vi "CmdConsole.Kill.vi"(8 "error in":errorcluster, 11 "CmdConsole in":refnum<class "CmdConsole.lvclass">) -> (0 "error out":errorcluster, 3 "CmdConsole out":refnum<class "CmdConsole.lvclass">)   [LabVIEW 2018, in "CmdConsole.lvclass"]
uses:
  CmdConsole.lvclass
  CmdConsole.lvclass/CmdConsole.ctl
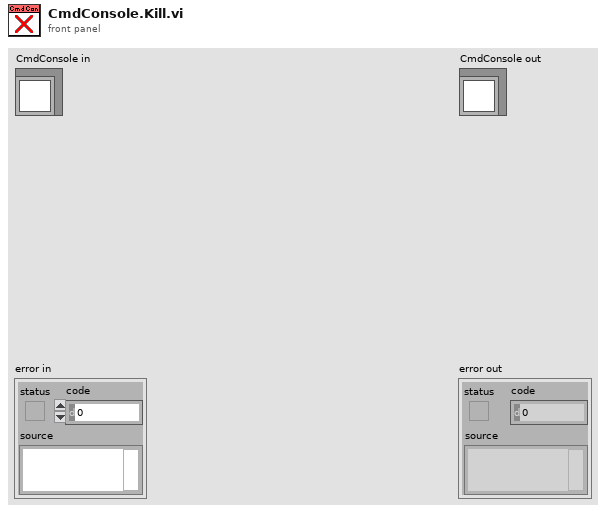
[diagram p1: front panel]
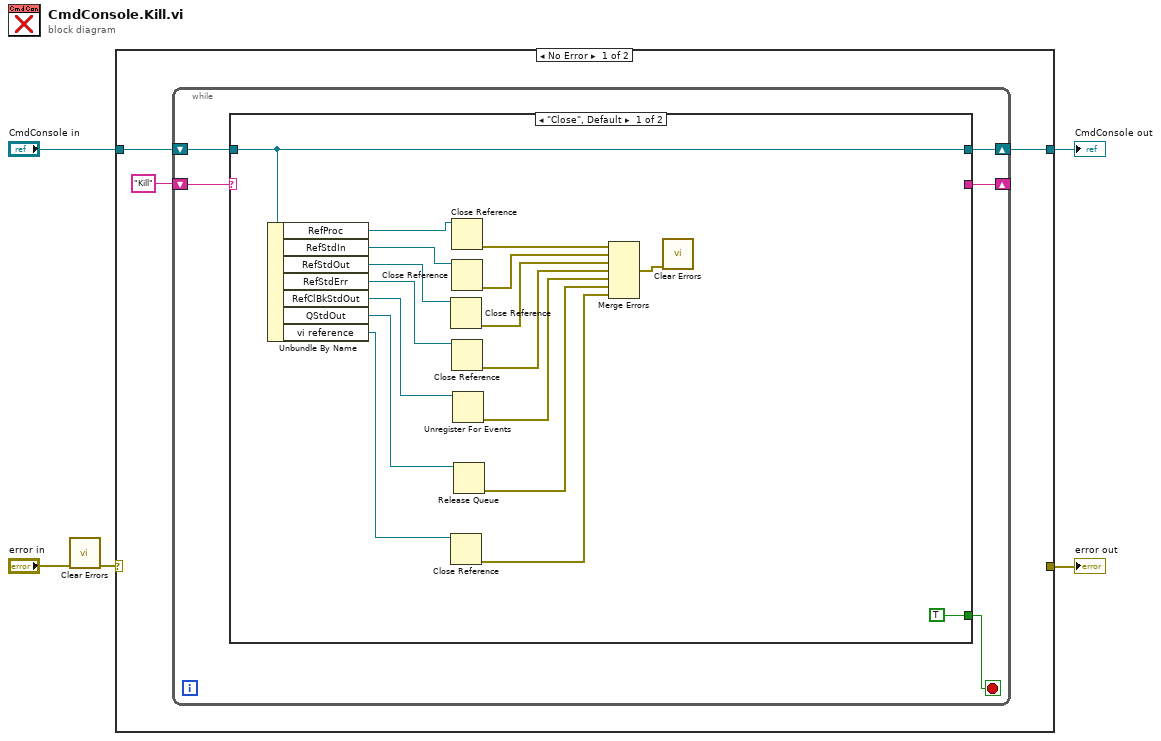
[diagram p0: block diagram]
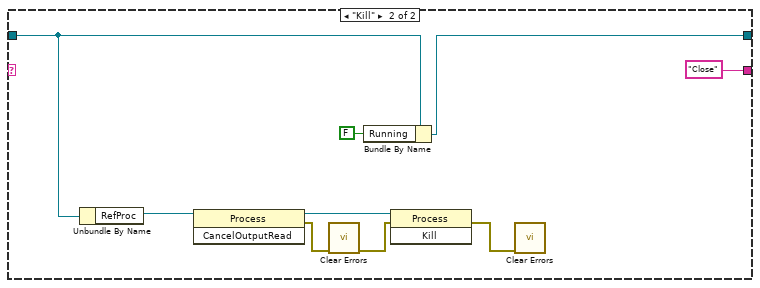
[diagram p2: hidden frame]
diagram:
  n1 = call <vilib>:"Clear Errors.vi"("error in (no error)"="error in") -> ("error out"=w2:errorcluster)  [unwired: 5 in, 1 out]
  n2 = case shown="No Error" w2 {
    selector: w2 -> [_ w41]
    tunnel: [_ w41] -> w5
    tunnel: [w7 w40] -> w3
    tunnel: "CmdConsole in" -> [w8 w40]
    frame No Error {
      n3 = while {
        shift-right: [w12] -> w7
        shift-left: w8 -> [w11]
        shift-right: [w13] -> _
        shift-left: "Kill" -> [w10]
        stop <- w9 stop-if-true
        n4 = case shown="\"Close\", Default" w10 {
          tunnel: w11 -> [w16 w33]
          tunnel: [_ "Close"] -> w13
          tunnel: [w16 w32] -> w12
          tunnel: [TRUE _] -> w9
          frame "Close", Default {
            n5 = Unbundle By Name(w16) -> ("RefProc"=w23:refnum<k24>, "RefStdIn"=w22:refnum<k24>, "RefStdOut"=w21:refnum<k24>, "RefStdErr"=w20:refnum<k24>, "RefClBkStdOut"=w19:refnum<k27>, "QStdOut"=w18:refnum<queue>, "vi reference"=w15:refnum<vi>)
            n6 = Close Reference(reference=w21) -> (error out=w27:errorcluster)  [unwired: 1 in]
            n7 = Close Reference(reference=w15) -> (error out=w14:errorcluster)  [unwired: 1 in]
            n8 = Close Reference(reference=w23) -> (error out=w29:errorcluster)  [unwired: 1 in]
            n9 = Close Reference(reference=w22) -> (error out=w28:errorcluster)  [unwired: 1 in]
            n10 = Close Reference(reference=w20) -> (error out=w26:errorcluster)  [unwired: 1 in]
            n11 = Unregister For Events(event registration refnum=w19) -> (error out=w24:errorcluster)  [unwired: 1 in]
            n12 = Release Queue(queue=w18) -> (error out=w17:errorcluster)  [unwired: 2 in, 2 out]
            n13 = Merge Errors(w29, w28, w27, w26, w24, w17, w14) -> (w25:errorcluster)
            n14 = call <vilib>:"Clear Errors.vi"("error in (no error)"=w25) -> ()  [unwired: 5 in, 2 out]
          }
          frame "Kill" {
            n15 = Unbundle By Name(w33) -> ("RefProc"=w39:refnum<k24>)
            n16 = invoke class="Process" method="CancelOutputRead"(reference=w39) -> (reference out=w38:refnum<k24>, error out=w37:errorcluster)  [unwired: 2 in, 1 out]
            n17 = call <vilib>:"Clear Errors.vi"("error in (no error)"=w37) -> ("error out"=w36:errorcluster)  [unwired: 5 in, 1 out]
            n18 = Bundle By Name(cluster=w33, "Running"=FALSE) -> (w32:refnum<class "CmdConsole.lvclass">)
            n19 = invoke class="Process" method="Kill"(reference=w38, error in=w36) -> (error out=w35:errorcluster)  [unwired: 1 in, 2 out]
            n20 = call <vilib>:"Clear Errors.vi"("error in (no error)"=w35) -> ()  [unwired: 5 in, 2 out]
          }
        }
      }
    }
    frame Error {
    }
  }
  "error out" <- w5
  "CmdConsole out" <- w3
